vi "PCO_Display.vi"() -> (1 "Raw_Length":u16, 4 "Length":u16, 6 "PCO_DisplayRaw_x64":T2, 7 "PCO_DisplayRaw_win32":T1, 8 "PCO_Display":T3)   [LabVIEW 2019, in "Convert.lvlib"]
doc: "Use this template to build a VI to use as a subVI."
uses:
  Convert.lvlib
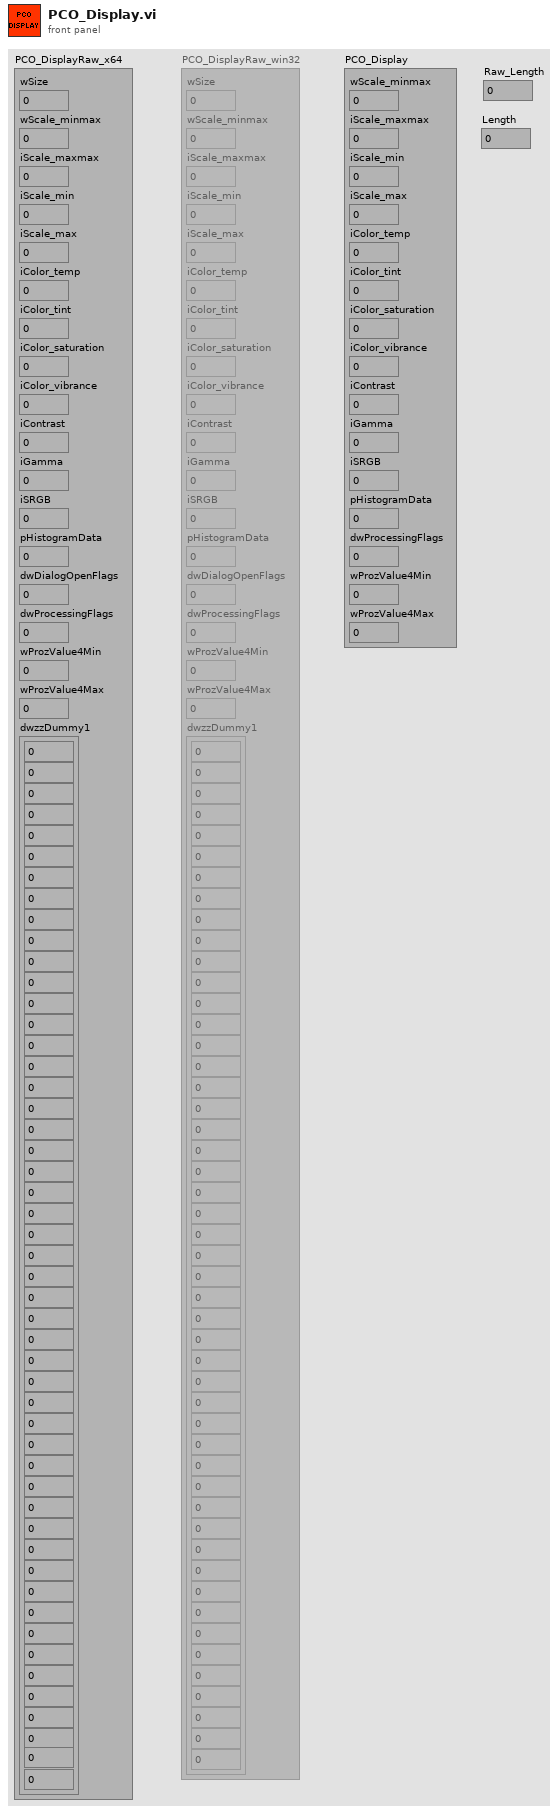
[diagram p1: front panel]
types:
  T1 = cluster{"wSize":u16, "wScale_minmax":u16, "iScale_maxmax":i32, "iScale_min":i32, "iScale_max":i32, "iColor_temp":i32, "iColor_tint":i32, "iColor_saturation":i32, "iColor_vibrance":i32, "iContrast":i32, "iGamma":i32, "iSRGB":i32, "pHistogramData":u32, "dwDialogOpenFlags":u32, "dwProcessingFlags":u32, "wProzValue4Min":u16, "wProzValue4Max":u16, "dwzzDummy1":cluster{u32, u32, u32, u32, u32, u32, u32, u32, u32, u32, u32, u32, u32, u32, u32, u32, u32, u32, u32, u32, u32, u32, u32, u32, u32, u32, u32, u32, u32, u32, u32, u32, u32, u32, u32, u32, u32, u32, u32, u32, u32, u32, u32, u32, u32, u32, u32, u32, u32}}
  T2 = cluster{"wSize":u16, "wScale_minmax":u16, "iScale_maxmax":i32, "iScale_min":i32, "iScale_max":i32, "iColor_temp":i32, "iColor_tint":i32, "iColor_saturation":i32, "iColor_vibrance":i32, "iContrast":i32, "iGamma":i32, "iSRGB":i32, "pHistogramData":u64, "dwDialogOpenFlags":u32, "dwProcessingFlags":u32, "wProzValue4Min":u16, "wProzValue4Max":u16, "dwzzDummy1":cluster{u32, u32, u32, u32, u32, u32, u32, u32, u32, u32, u32, u32, u32, u32, u32, u32, u32, u32, u32, u32, u32, u32, u32, u32, u32, u32, u32, u32, u32, u32, u32, u32, u32, u32, u32, u32, u32, u32, u32, u32, u32, u32, u32, u32, u32, u32, u32, u32, u32, u32}}
  T3 = cluster{"wScale_minmax":u16, "iScale_maxmax":i32, "iScale_min":i32, "iScale_max":i32, "iColor_temp":i32, "iColor_tint":i32, "iColor_saturation":i32, "iColor_vibrance":i32, "iContrast":i32, "iGamma":i32, "iSRGB":i32, "pHistogramData":u64, "dwProcessingFlags":u32, "wProzValue4Min":u16, "wProzValue4Max":u16}
  T4 = cluster{u32, u32, u32, u32, u32, u32, u32, u32, u32, u32, u32, u32, u32, u32, u32, u32, u32, u32, u32, u32, u32, u32, u32, u32, u32, u32, u32, u32, u32, u32, u32, u32, u32, u32, u32, u32, u32, u32, u32, u32, u32, u32, u32, u32, u32, u32, u32, u32, u32, u32}
  T5 = cluster{u32, u32, u32, u32, u32, u32, u32, u32, u32, u32, u32, u32, u32, u32, u32, u32, u32, u32, u32, u32, u32, u32, u32, u32, u32, u32, u32, u32, u32, u32, u32, u32, u32, u32, u32, u32, u32, u32, u32, u32, u32, u32, u32, u32, u32, u32, u32, u32, u32}
  T6 = enum8{"Enabled", "Disabled", "Disabled and Grayed Out"}
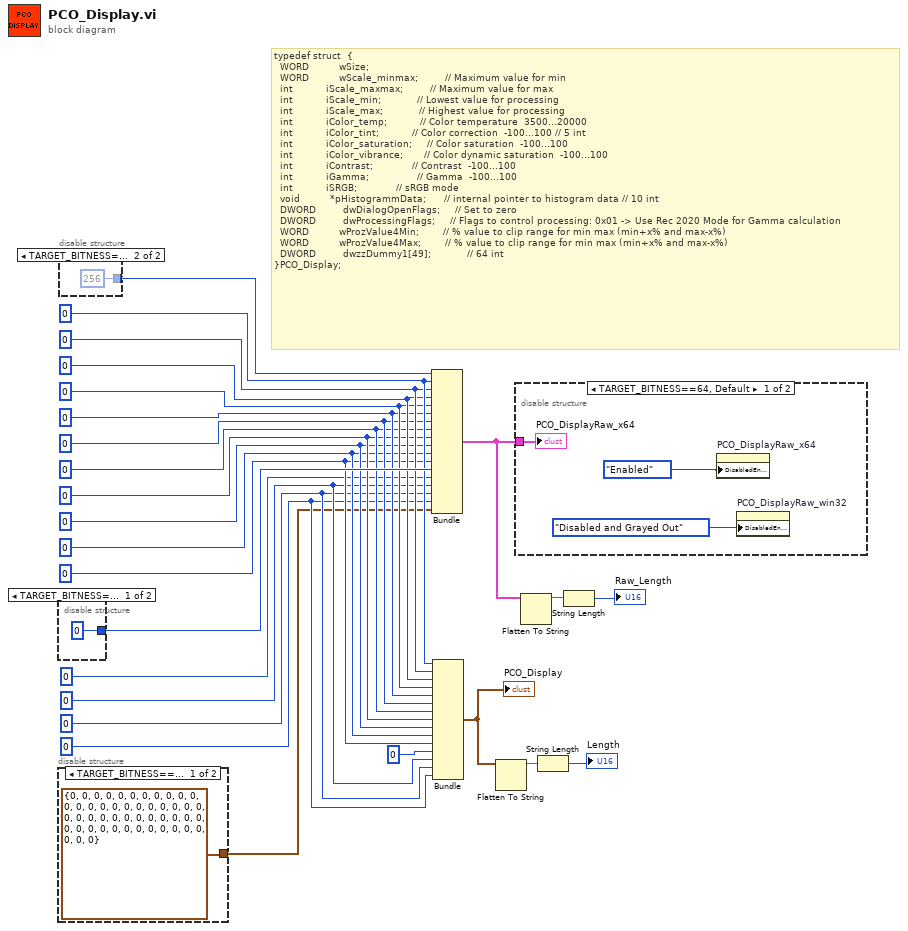
[diagram p0: block diagram]
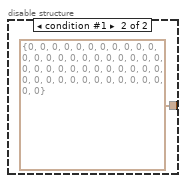
[diagram p2: hidden frame]
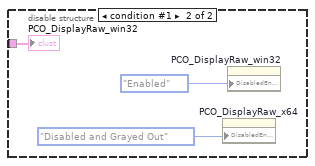
[diagram p3: hidden frame]
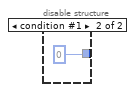
[diagram p4: hidden frame]
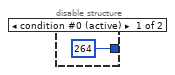
[diagram p5: hidden frame]
diagram:
  w2 = u16 0 ("wProzValue4Max")
  w3 = u16 0 ("wProzValue4Min")
  w4 = u32 0 ("dwProcessingFlags")
  w7 = 0 ("iSRGB")
  w8 = 0 ("iGamma")
  w9 = 0 ("iContrast")
  w10 = 0 ("iColor_vibrance")
  w11 = 0 ("iColor_saturation")
  w12 = 0 ("iColor_tint")
  w13 = 0 ("iColor_temp")
  w14 = 0 ("iScale_max")
  w15 = 0 ("iScale_min")
  w16 = 0 ("iScale_maxmax")
  w17 = u16 0 ("wScale_minmax")
  # "typedef struct  {\n  WORD          wSize;\n  WORD          wScale_minmax;         // Maximum value for min\n  int           iScale_maxmax;         // Maximum value for max \n  int           iScale_min;            // Lowest value for processing\n  int           iScale_max;            // Highest value for processing\n  int           iColor_temp;           // Color temperature  3500...20000\n  int           iColor_tint;           // Color correction  -100...100 // 5 int\n  int           iColor_saturation;     // Color saturation  -100...100\n  int           iColor_vibrance;       // Color dynamic saturation  -100...100\n  int           iContrast;             // Contrast  -100...100\n  int           iGamma;                // Gamma  -100...100\n  int           iSRGB;\t\t\t\t         // sRGB mode\n  void          *pHistogrammData;      // internal pointer to histogram data // 10 int\n  DWORD         dwDialogOpenFlags;     // Set to zero\n  DWORD         dwProcessingFlags;     // Flags to control processing: 0x01 -> Use Rec 2020 Mode for Gamma calculation\n  WORD          wProzValue4Min;        // % value to clip range for min max (min+x% and max-x%) \n  WORD          wProzValue4Max;        // % value to clip range for min max (min+x% and max-x%) \n  DWORD         dwzzDummy1[49];            // 64 int\n}PCO_Display;"
  n1 = disable-structure "Diagram Disable Structure" shown="TARGET_BITNESS==64, Default" {
    disable-tunnel: [u64 0 ("pHistogramData") u32 0 ("pHistogramData")] -> w19
    frame condition #0 (active) {
    }
    frame condition #1 {
    }
  }
  n2 = disable-structure "Diagram Disable Structure" shown="TARGET_BITNESS==64, Default" {
    disable-tunnel: [T4 {0, 0, 0, 0, 0, 0, 0, 0, 0, 0, 0, 0, 0, 0, 0, 0, 0, 0, 0, 0, 0, 0, 0, 0, 0, 0, 0, 0, 0, 0, 0, 0, 0, 0, 0, 0, 0, 0, 0, 0, 0, 0, 0, 0, 0, 0, 0, 0, 0, 0} ("dwzzDummy1") T5 {0, 0, 0, 0, 0, 0, 0, 0, 0, 0, 0, 0, 0, 0, 0, 0, 0, 0, 0, 0, 0, 0, 0, 0, 0, 0, 0, 0, 0, 0, 0, 0, 0, 0, 0, 0, 0, 0, 0, 0, 0, 0, 0, 0, 0, 0, 0, 0, 0} ("dwzzDummy1")] -> w1
    frame condition #0 (active) {
    }
    frame condition #1 {
    }
  }
  n3 = disable-structure "Diagram Disable Structure" shown="TARGET_BITNESS==32" {
    disable-tunnel: [u16 264 ("wSize") u16 256 ("wSize")] -> w20
    frame condition #0 (active) {
    }
    frame condition #1 {
    }
  }
  n4 = Bundle("wSize"=w20, "wScale_minmax"=w17, "iScale_maxmax"=w16, "iScale_min"=w15, "iScale_max"=w14, "iColor_temp"=w13, "iColor_tint"=w12, "iColor_saturation"=w11, "iColor_vibrance"=w10, "iContrast"=w9, "iGamma"=w8, "iSRGB"=w7, "pHistogramData"=w19, "dwDialogOpenFlags"=u32 0, "dwProcessingFlags"=w4, "wProzValue4Min"=w3, "wProzValue4Max"=w2, "dwzzDummy1"=w1) -> (w18:T2)  [unwired: 1 in]
  n5 = Bundle("wScale_minmax"=w17, "iScale_maxmax"=w16, "iScale_min"=w15, "iScale_max"=w14, "iColor_temp"=w13, "iColor_tint"=w12, "iColor_saturation"=w11, "iColor_vibrance"=w10, "iContrast"=w9, "iGamma"=w8, "iSRGB"=w7, "pHistogramData"=u64 0, "dwProcessingFlags"=w4, "wProzValue4Min"=w3, "wProzValue4Max"=w2) -> (w25:T3)  [unwired: 1 in]
  "PCO_Display" <- w25
  n6 = Flatten To String(anything=w25) -> (data string=w24:string)  [unwired: 3 in, 2 out]
  n7 = disable-structure "Diagram Disable Structure" shown="TARGET_BITNESS==64, Default" {
    disable-tunnel: w18 -> [w34 w36]
    frame condition #0 (active) {
      n8 = property on="PCO_DisplayRaw_x64" class="Clust (strict)"("DisabledEnum"=T6."Enabled" ("Disabled")) -> ()  [unwired: 2 in, 2 out]
      n9 = property on="PCO_DisplayRaw_win32" class="Clust (strict)"("DisabledEnum"=T6."Disabled and Grayed Out" ("Disabled")) -> ()  [unwired: 2 in, 2 out]
      "PCO_DisplayRaw_x64" <- w34
    }
    frame condition #1 {
      n10 = property on="PCO_DisplayRaw_x64" class="Clust (strict)"("DisabledEnum"=T6."Disabled and Grayed Out" ("Disabled")) -> ()  [unwired: 2 in, 2 out]
      n11 = property on="PCO_DisplayRaw_win32" class="Clust (strict)"("DisabledEnum"=T6."Enabled" ("Disabled")) -> ()  [unwired: 2 in, 2 out]
      "PCO_DisplayRaw_win32" <- w36
    }
  }
  n12 = Flatten To String(anything=w18) -> (data string=w23:string)  [unwired: 3 in, 2 out]
  n13 = String Length(string=w24) -> (length=→"Length":i32)
  n14 = String Length(string=w23) -> (length=→"Raw_Length":i32)
